vi "Get ClassName From Flattened Object.vi"(5 "Read String (T)":bool=TRUE, 11 "Flattened Object Data":u8[](array[numeric])) -> (1 "Index After ClassName":i32, 2 "Class Name":string)   [LabVIEW 2017, in "Composition.lvlib"]
doc: "Gets the class name from flattened object data."
uses:
  Composition.lvlib
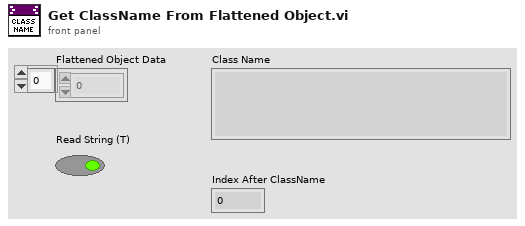
[diagram p1: front panel]
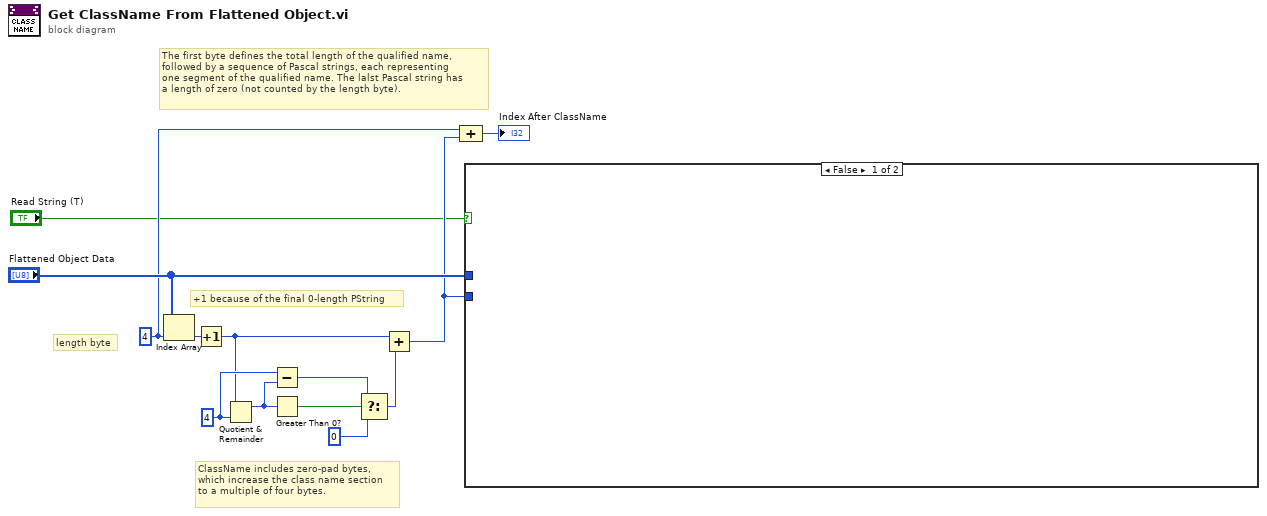
[diagram p0: block diagram]
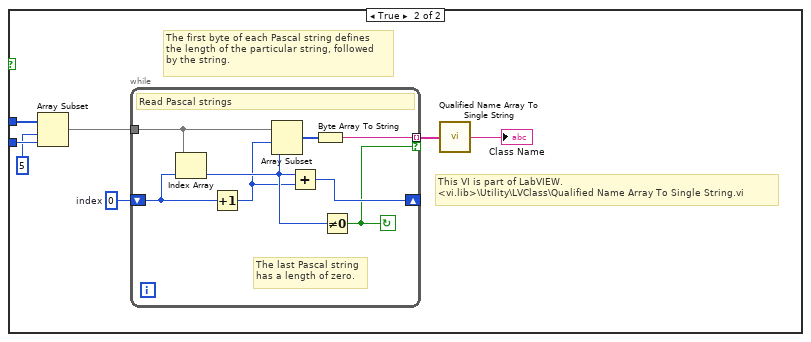
[diagram p2: hidden frame]
diagram:
  w3 = 4 ("index")
  w13 = u8 4 ("y")
  # "+1 because of the final 0-length PString"
  # "ClassName includes zero-pad bytes,\nwhich increase the class name section\nto a multiple of four bytes."
  # "length byte"
  # "The first byte defines the total length of the qualified name,\nfollowed by a sequence of Pascal strings, each representing\none segment of the qualified name. The lalst Pascal string has\na length of zero (not counted by the length byte)."
  n1 = Index Array(array="Flattened Object Data", index=w3) -> (element=w9:u8)
  n2 = Increment(x=w9) -> (x+1=w2:u8)
  n3 = Quotient & Remainder(x=w2, y=w13) -> (x-y*floor(x/y)=w12:u8)  [unwired: 1 out]
  n4 = Subtract(x=w13, y=w12) -> (x-y=w6:u8)
  n5 = Greater Than 0?(x=w12) -> (x > 0?=w11:bool)
  n6 = Select(t=w6, s=w11, f=u8 0 ("t")) -> (s? t:f=w10:u8)
  n7 = Add(x=w2, y=w10) -> (x+y=w4:u8)
  n8 = Compound Arithmetic op=unknown(w3, w4) -> (→"Index After ClassName":i32)
  n9 = case shown="False" "Read String (T)" {
    tunnel: "Flattened Object Data" -> [_ w16]
    tunnel: w4 -> [_ w15]
    frame False {
    }
    frame True {
      w20 = 0  # index
      # "This VI is part of LabVIEW.\n<vi.lib>\\Utility\\LVClass\\Qualified Name Array To Single String.vi"
      # "The first byte of each Pascal string defines\nthe length of the particular string, followed\nby the string."
      n10 = Array Subset(array=w16, index=5, length=w15) -> (w19:u8[])
      n11 = while {
        tunnel: w19 -> [w28]
        shift-right: [w26] -> _
        shift-left: w20 -> [w25]
        tunnel: [w23] -> w18 mode=indexing if=w21
        stop <- w21 continue-if-true
        # "The last Pascal string\nhas a length of zero."
        # "Read Pascal strings"
        n12 = Index Array(array=w28, index=w25) -> (element=w24:u8)
        n13 = Increment(x=w25) -> (x+1=w22:i32)
        n14 = Array Subset(array=w28, index=w22, length=w24) -> (w27:u8[])
        n15 = Add(x=w24, y=w22) -> (x+y=w26:i32)
        n16 = Byte Array To String(unsigned byte array=w27) -> (string=w23:string)
        n17 = Not Equal To 0?(x=w24) -> (x != 0?=w21:bool)
      }
      n18 = call <vilib>:"Qualified Name Array To Single String.vi"("Fully Qualified Array"=w18) -> ("Fully Qualified String"=→"Class Name":string)
    }
  }
